vi "program seq..vi"(6 "IOList":T3, 7 "Cluster data":T5, 11 "Filepath":path=path "E:/My Project/2018-2019/Under development/Minda Ind. Switch -ID 144-145/Project/data/trail pro -12.txt") -> (0 "Error Out":errorcluster)   [LabVIEW 2015]
uses:
  Control PB/Active.ctl
  Control PB/deactive.ctl
  Control PB/output control.ctl
  Control PB/input control.ctl
  Control PB/timer.ctl
  Control PB/Remove list.ctl
  Control Button/Exit.ctl
  Control PB/Add_s.ctl
  Control PB/Delete_.ctl
  Control Button/Save.ctl
  Control PB/motor.ctl
  Control PB/Camera.ctl
  Control PB/Barcode.ctl
  Galobal variable_TI.vi
panel:
  out "Step List 4":string[](array[string])
  out "Step List 3":string[](array[string])
  in  "Barcode":T1
  in  "Camera":T2
  out "x <= y?":bool
  out "Cancel":bool
  out "Step List 2":string[](array[string])
  out "Pokayoka Result":cluster{"Sensor Name":string, "Boolean":bool}[](array[cluster])
  in  "Feed Back Channel":i32[](listbox)=[0]
  out "Input":bool[](array[boolean])
  out "Feature List (Out) 2":T4(array[cluster])
  out "error out 2":errorcluster
  in  "Control":bool
  out "Station No":string
  out "Model Name":string
  out "Machine Name":string
  in  "Motor":T6
  in  "Feature List":i32(listbox) caption="Steps List"
  in  "Deletefeature list":T7
  in  "Add feature list":T8
  in  "Deactive":T9
  in  "Active":T10
  in  "Program step":i32(listbox)
  in  "Remove Step":T11
  in  "Wait Time":u32=100 caption="Timer(ms)" max=600000 step=1
  in  "Timer":T12
  in  "Save":T13
  in  "stop":T14
  in  "op Add":T15
  in  "Input Add":T16
  out "Step List":string[](array[string])
  out "output cluster":T17
  in  "Analog":bool
  in  "Analog Input":i32[](listbox)=[0]
  in  "Control Channel":i32[](listbox)=[7]
  in  "Steps":T18(array[cluster])
  in  "Program mode":string="Data"
  out "error out":errorcluster
  out "Feature List (Out)":T19(array[cluster])
  # "Program Sequence Window"
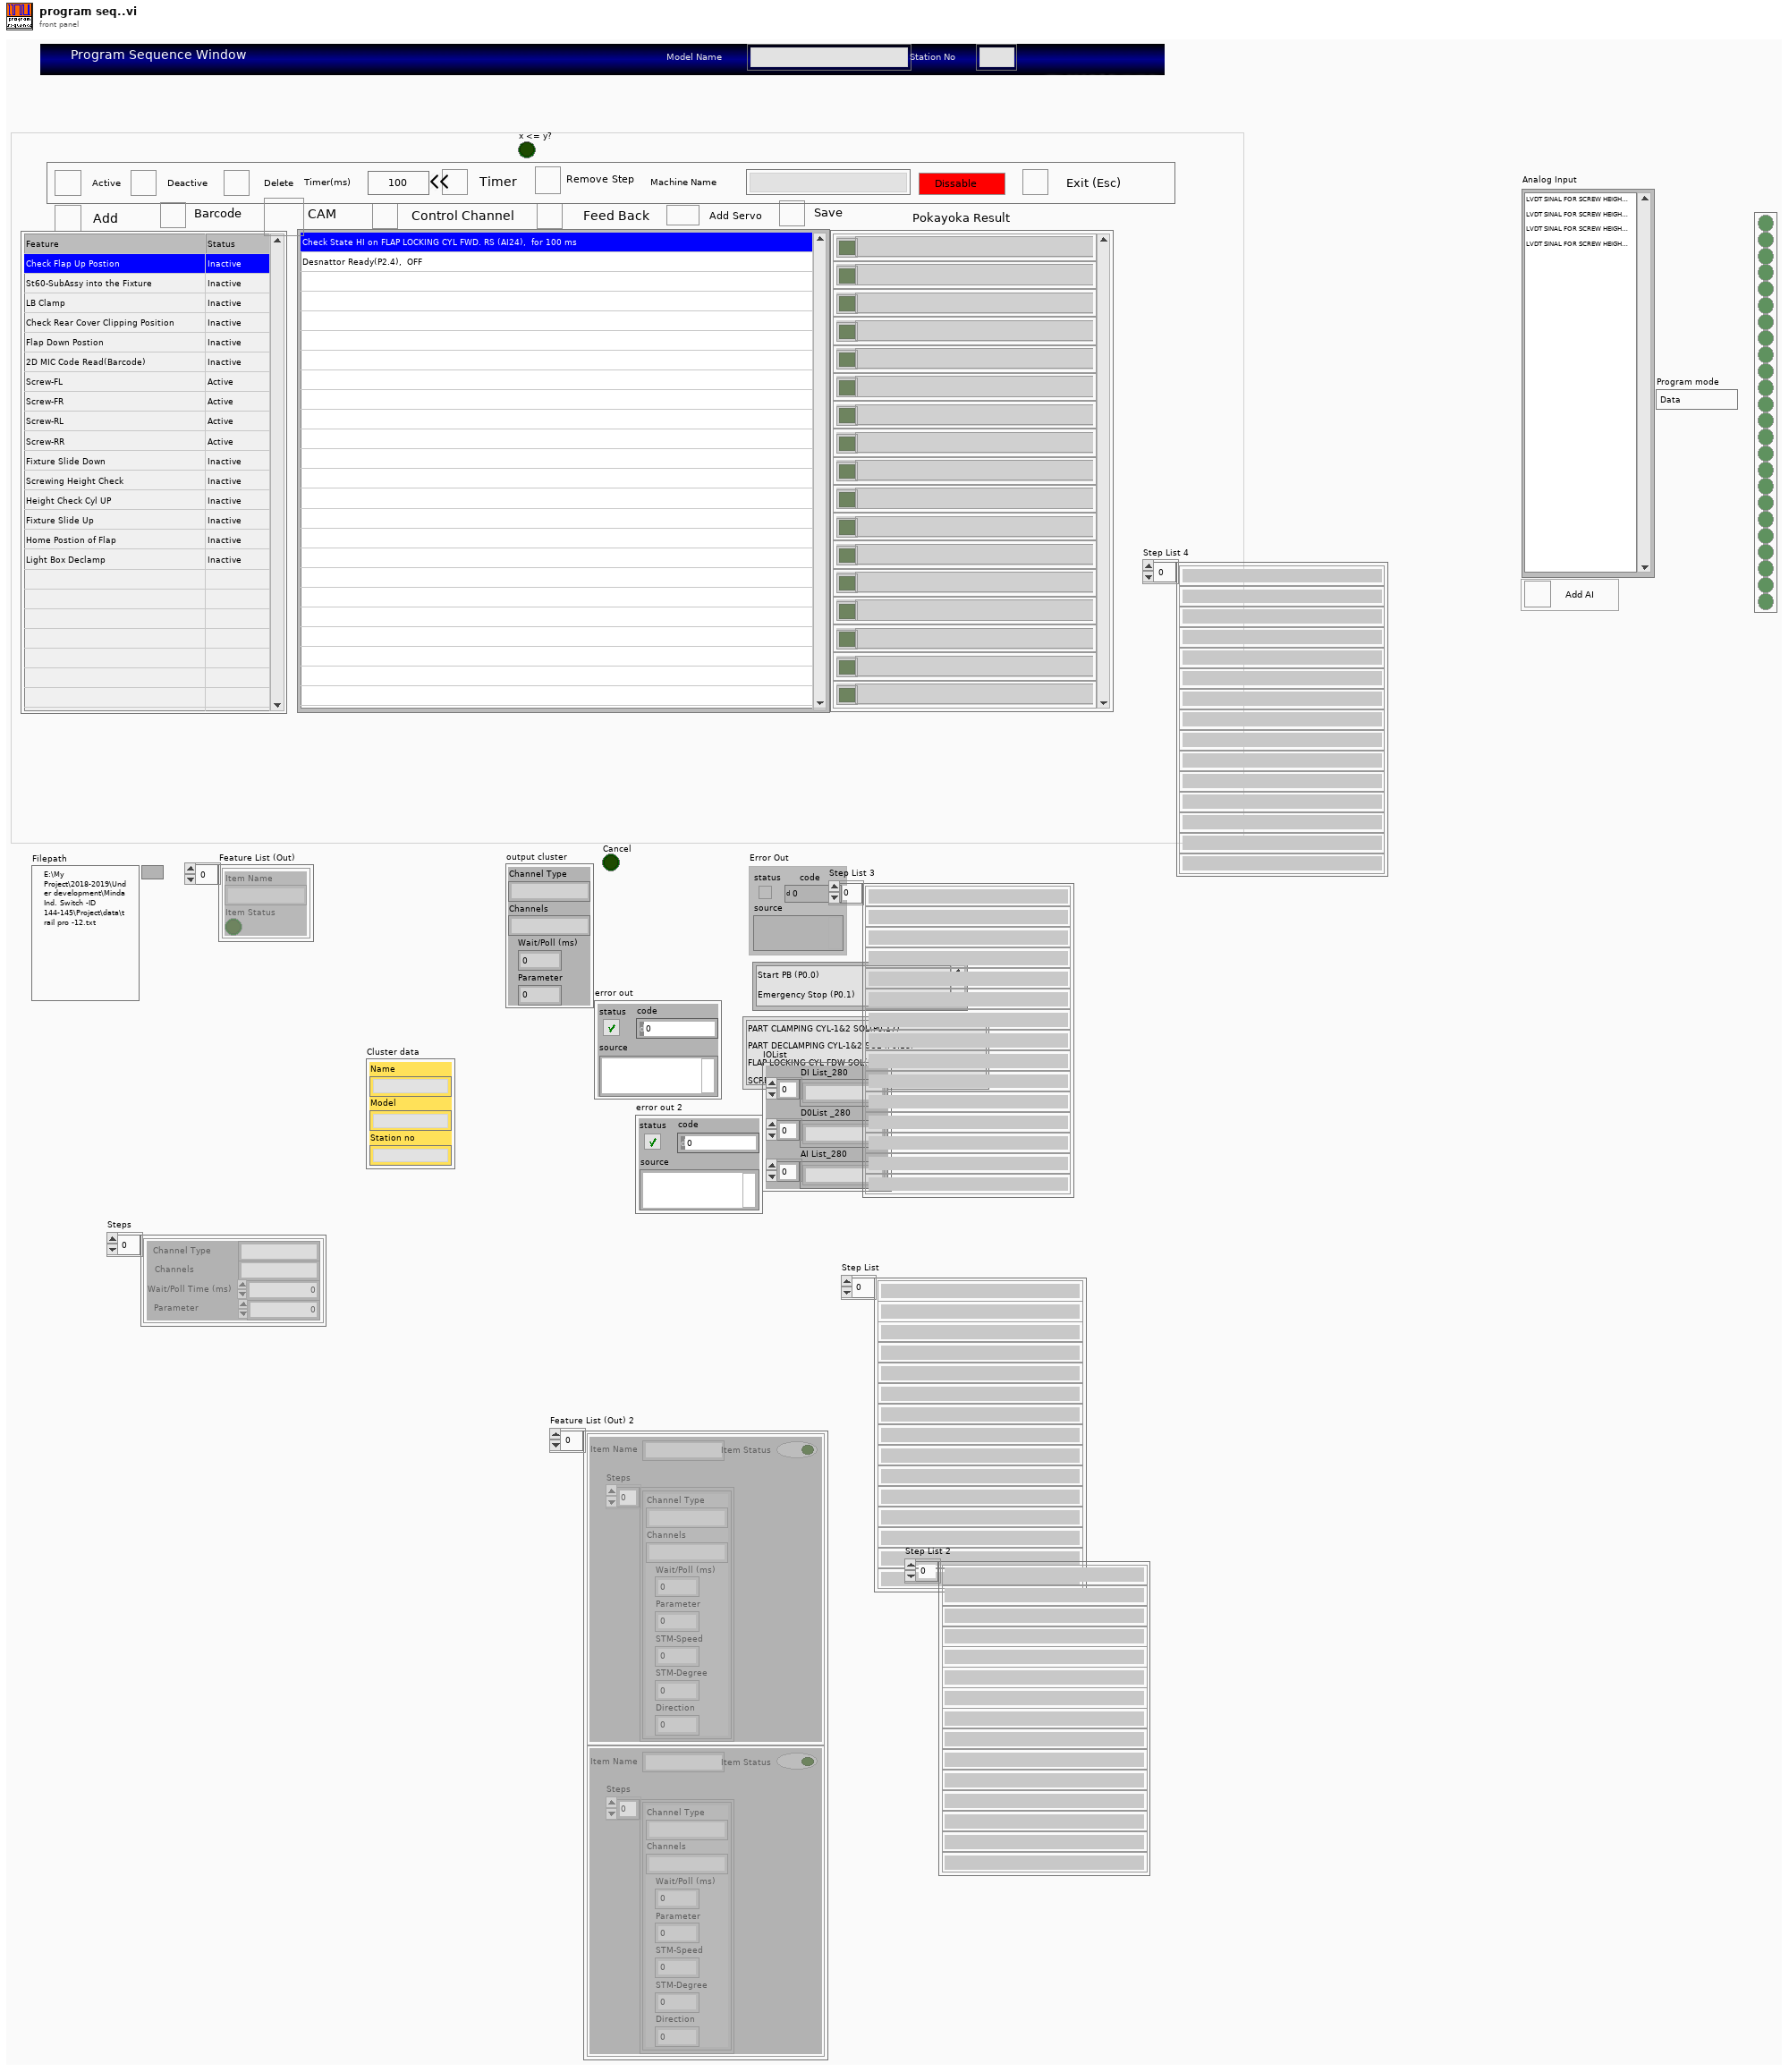
[diagram p1: front panel]
types:
  T1 = typedef "Barcode.ctl" = bool
  T2 = typedef "Camera.ctl" = bool
  T3 = cluster{"DI List_280":string[], "D0List _280":string[], "AI List_280":string[]}
  T4 = cluster{"Item Name":string, "Item Status":bool, "Steps":cluster{"Channel Type":string, "Channels":string, "Wait/Poll (ms)":u32, "Parameter":u8, "STM-Speed":i32, "STM-Degree":u32, "Direction":u8}[]}[]
  T5 = cluster{"Name":string, "Model":string, "Station no":string}
  T6 = typedef "motor.ctl" = bool
  T7 = typedef "Delete_.ctl" = bool
  T8 = typedef "Add_s.ctl" = bool
  T9 = typedef "deactive.ctl" = bool
  T10 = typedef "Active.ctl" = bool
  T11 = typedef "Remove list.ctl" = bool
  T12 = typedef "timer.ctl" = bool
  T13 = typedef "Save.ctl" = bool
  T14 = typedef "Exit.ctl" = bool
  T15 = typedef "output control.ctl" = bool
  T16 = typedef "input control.ctl" = bool
  T17 = cluster{"Channel Type":string, "Channels":string, "Wait/Poll (ms)":u32, "Parameter":u8}
  T18 = cluster{"Channel Type":string, "Channels":string, "Wait/Poll Time (ms)":u32, "Parameter":u8}[]
  T19 = cluster{"Item Name":string, "Item Status":bool}[]
  T20 = cluster{"Channel Type":string, "Channels":string, "Wait/Poll (ms)":u32, "Parameter":u8, "STM-Speed":i32, "STM-Degree":i32, "Direction":u8}
  T21 = cluster{"Item Name":string, "Item Status":bool, "Steps":cluster{"Channel Type":string, "Channels":string, "Wait/Poll (ms)":u32, "Parameter":u8, "STM-Speed":i32, "STM-Degree":u32, "Direction":u8}[]}
  T22 = cluster{"Channel Type":string, "Channels":string, "Wait/Poll (ms)":u32, "Parameter":u8, "STM-Speed":i32, "STM-Degree":u32, "Direction":u8}[]
  T23 = cluster{"Item Name":string, "Active":T10, "Steps":cluster{"Channel Type":string, "Channels":string, "Wait/Poll (ms)":u32, "Parameter":u8, "STM-Speed":i32, "STM-Degree":u32, "Direction":u8}[]}
  T24 = cluster{"Channel Type":string, "Channels":string, "Wait/Poll (ms)":u32, "Parameter":u8, "STM-Speed":i32, "STM-Degree":i32, "Direction":u8}[]
  T25 = cluster{"Feature name ":string, bool, cluster{"Channel Type":string, "Channels":string, "Wait/Poll (ms)":u32, "Parameter":u8, "STM-Speed":i32, "STM-Degree":i32, "Direction":u8}[]}
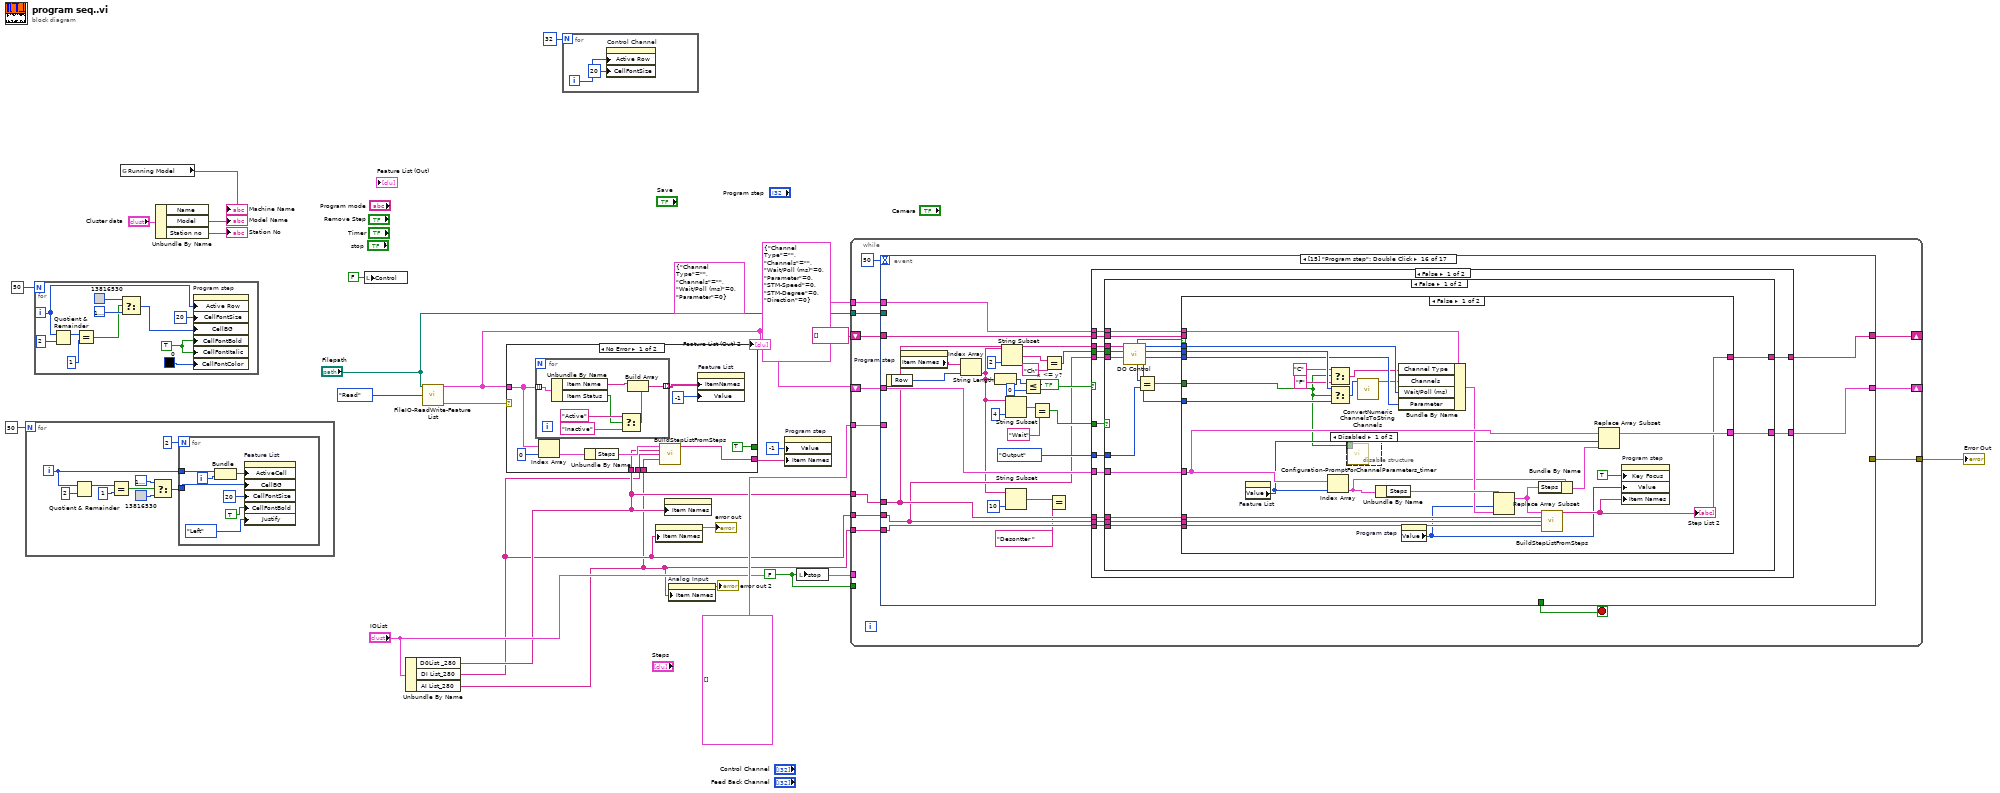
[diagram p0: block diagram]
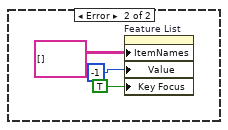
[diagram p2: hidden frame]
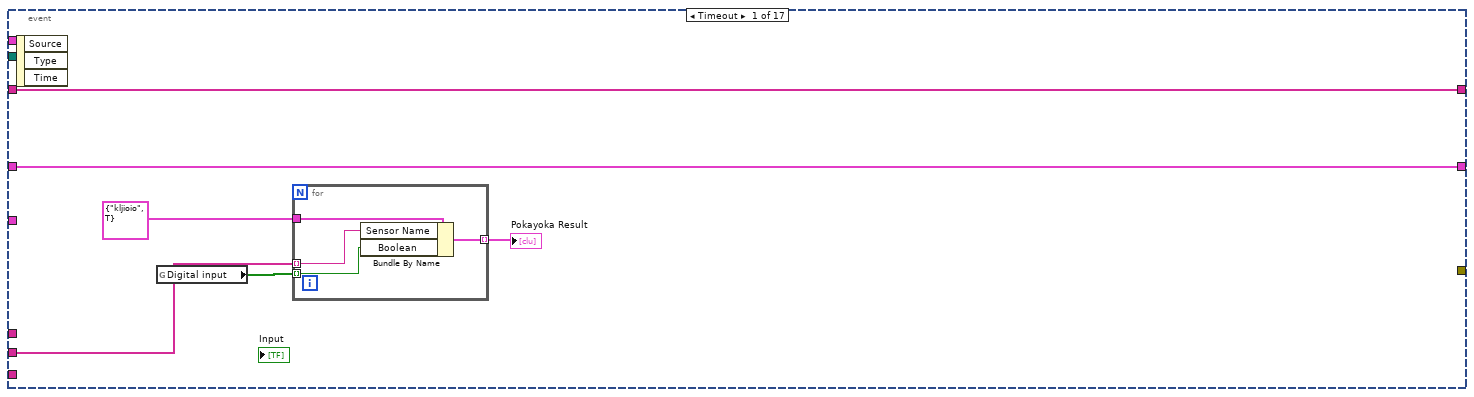
[diagram p3: hidden frame]
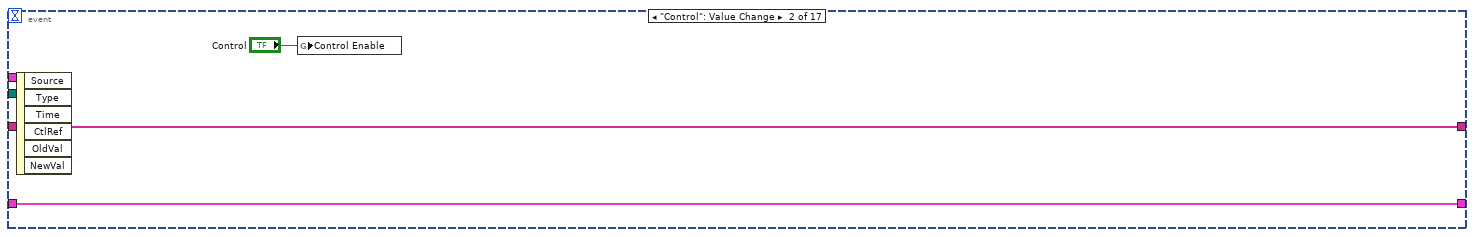
[diagram p4: hidden frame]
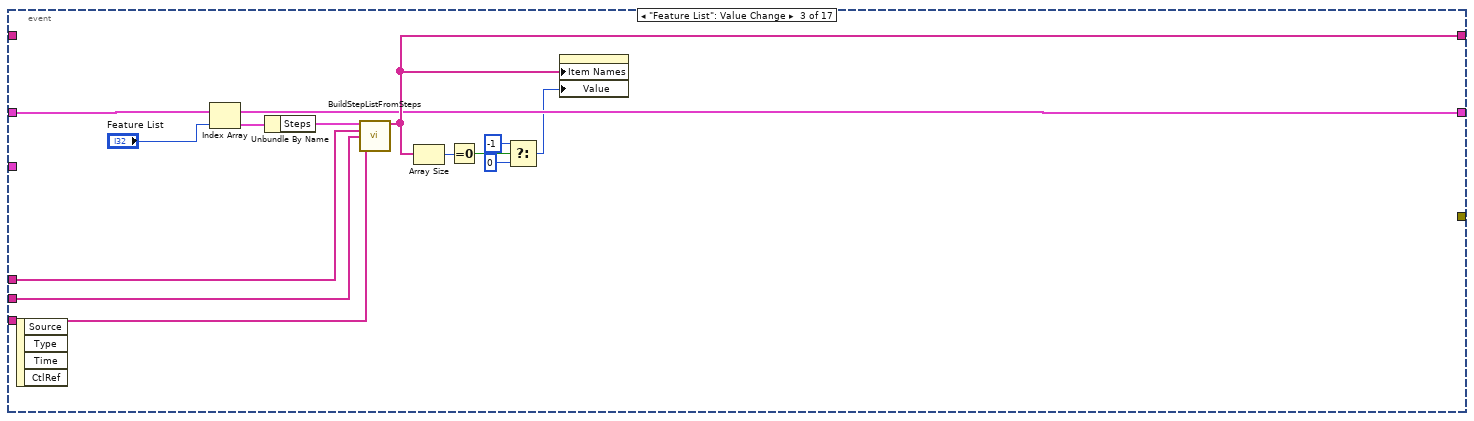
[diagram p5: hidden frame]
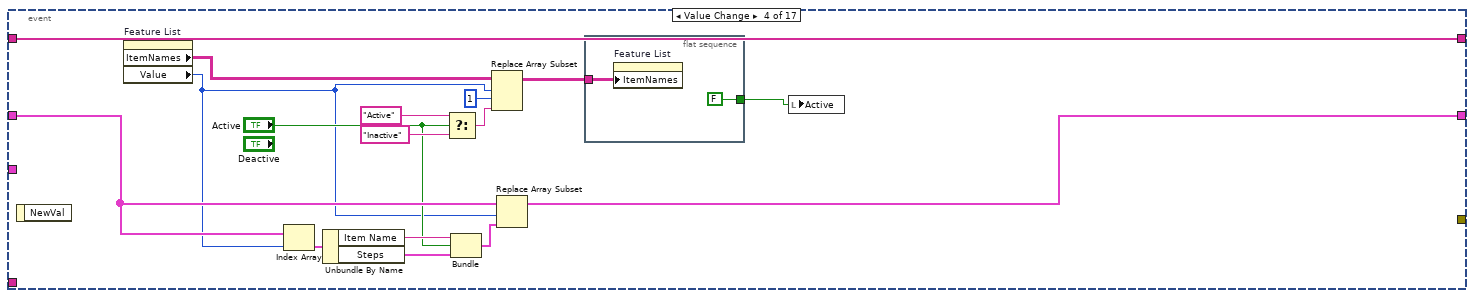
[diagram p6: hidden frame]
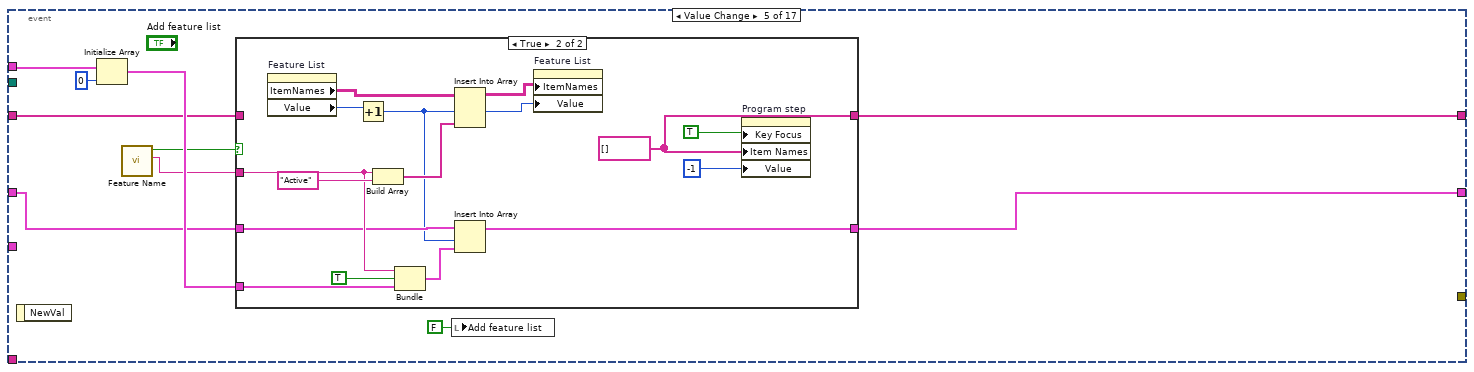
[diagram p7: hidden frame]
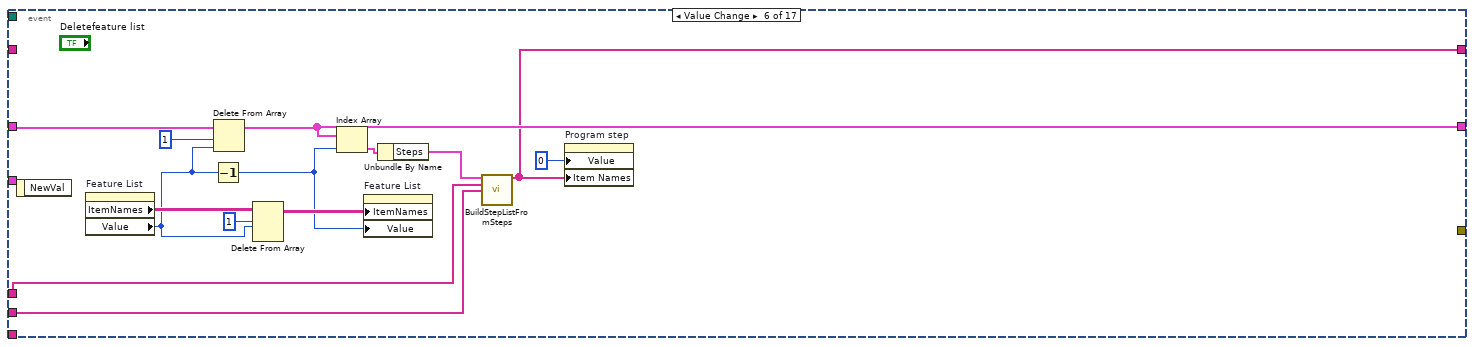
[diagram p9: hidden frame]
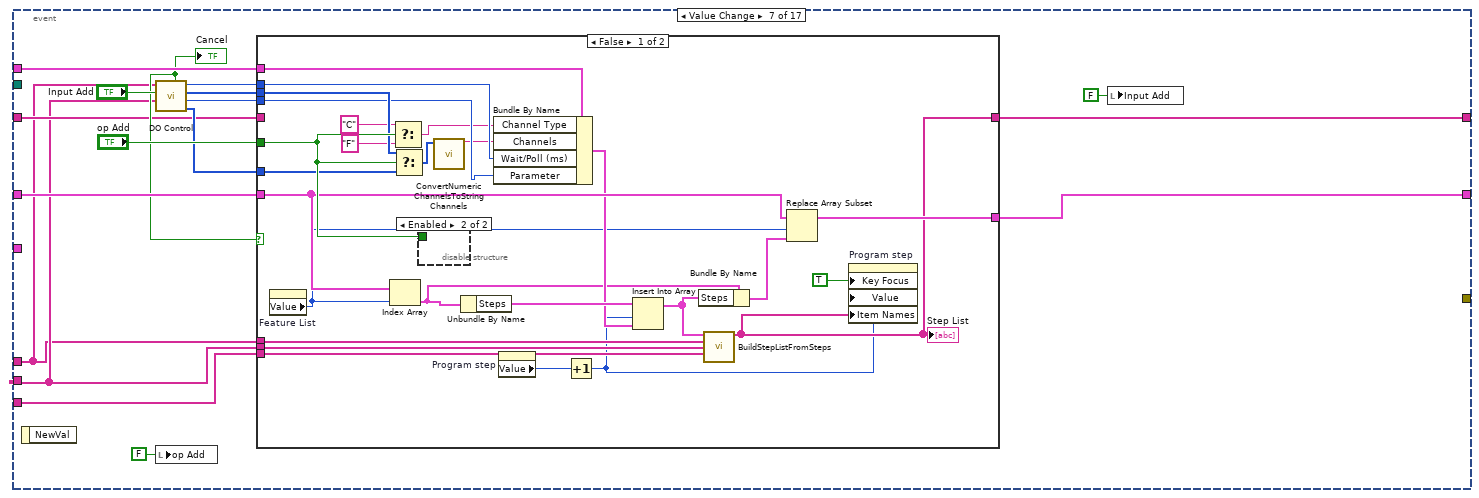
[diagram p10: hidden frame]
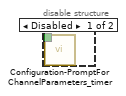
[diagram p11: hidden frame]
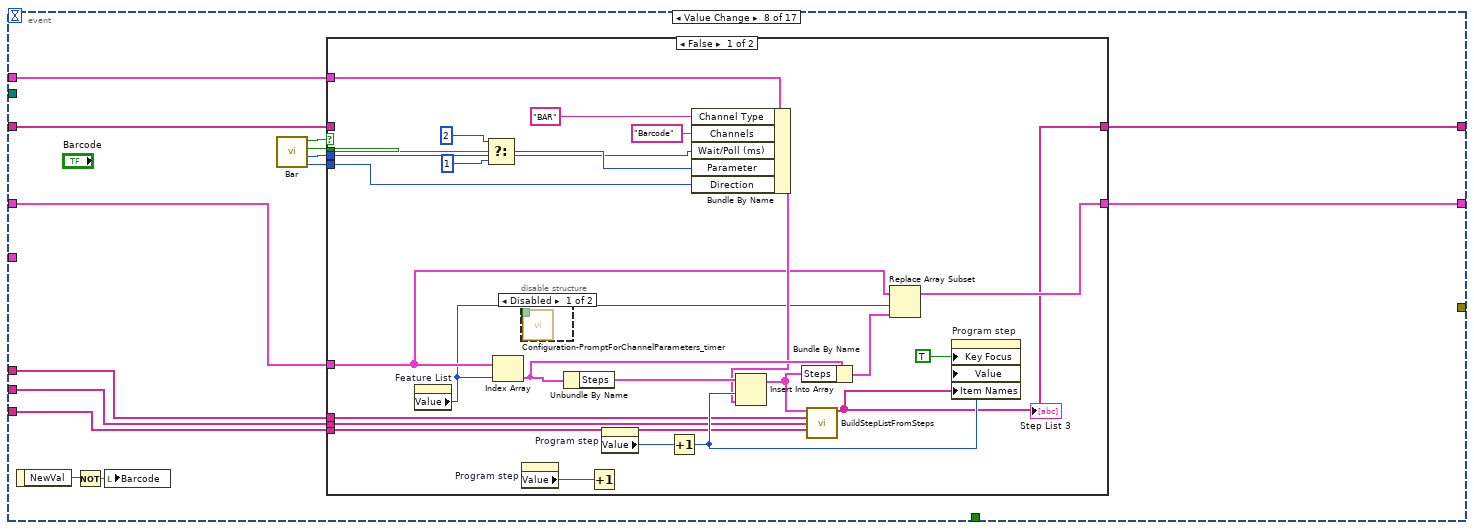
[diagram p13: hidden frame]
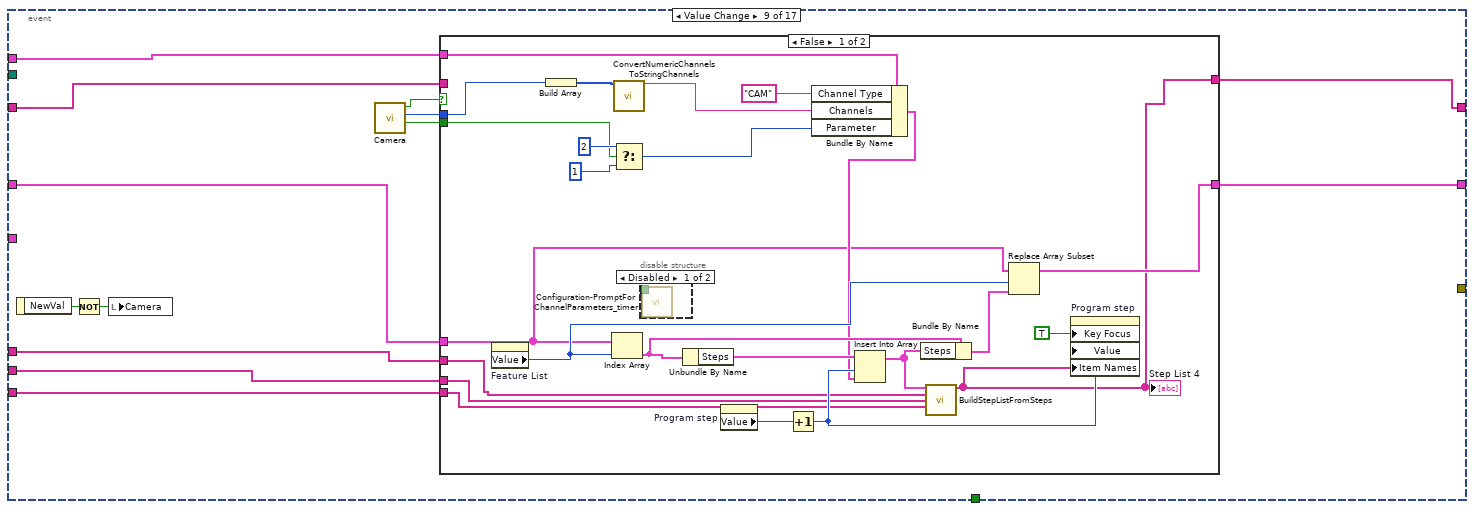
[diagram p16: hidden frame]
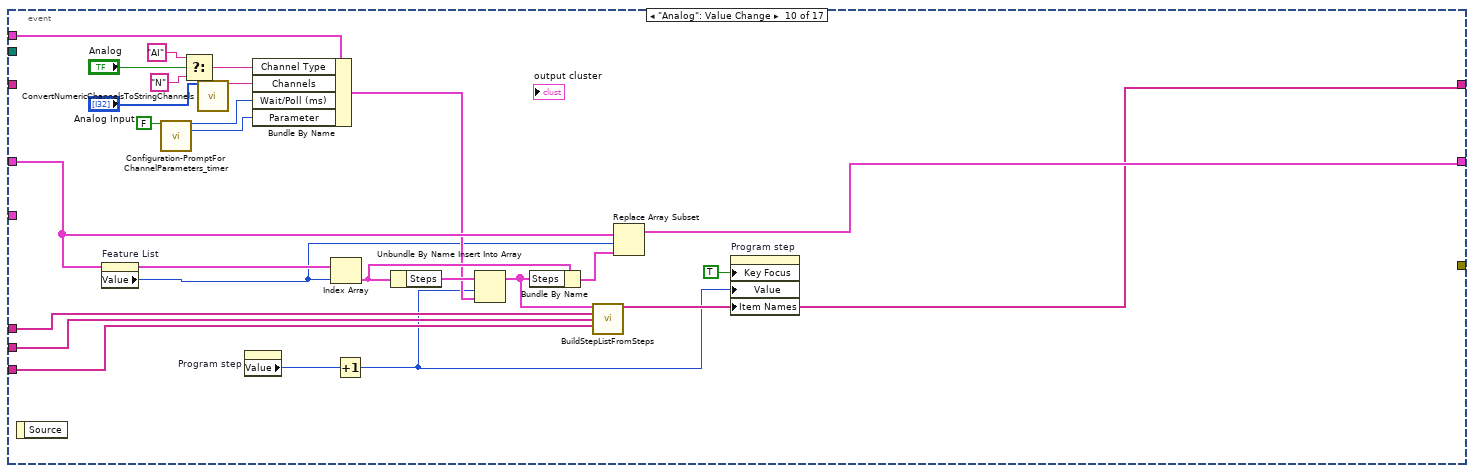
[diagram p19: hidden frame]
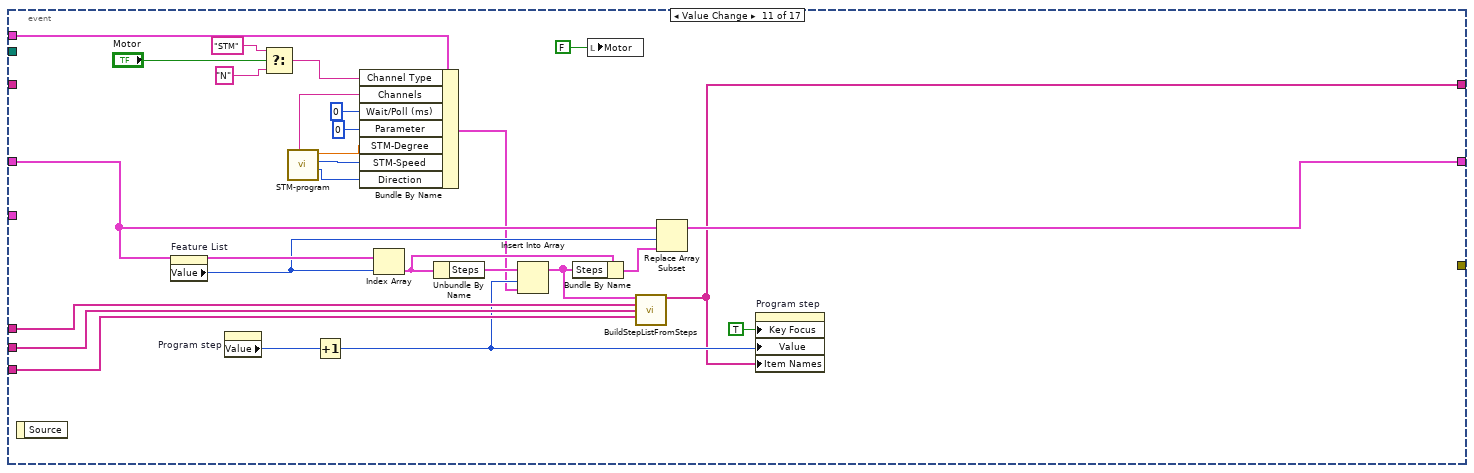
[diagram p20: hidden frame]
diagram:
  w9 = FALSE ("stop")
  (unwired) T17 {"Channel Type"="", "Channels"="", "Wait/Poll (ms)"=0, "Parameter"=0} ("Step")
  n1 = for {
    N: 50 -> [_]
    i -> [w33]
    n2 = Quotient & Remainder(x=w33, y=2) -> (x-y*floor(x/y)=w31:i32)  [unwired: 1 out]
    n3 = Equal?(x=w31, y=1) -> (x = y?=w29:bool)
    n4 = Select(t=u32 16777225 ("Color Box"), s=w29, f=u32 13816530 ("Color Box")) -> (s? t:f=w26:u32)
    n5 = for {
      N: 2 -> [_]
      tunnel: w33 -> [w41]
      tunnel: w26 -> [w38]
      i -> [w40]
      n6 = Bundle(w41, w40) -> (w39:cluster{i32, i32})  [unwired: 1 in]
      n7 = property on="Feature List" class="MCListbox (strict)"("ActiveCell"=w39, "CellBG"=w38, "CellFontSize"=u32 20 ("Active Cell:Cell Font:Size"), "CellFontBold"=TRUE ("Active Cell:Cell Font:Bold"), "Justify"=enum16{"Left", "Center", "Right"}."Left" ("Active Cell:Cell Justification")) -> ()  [unwired: 2 in, 2 out]
    }
  }
  n8 = for {
    N: 50 -> [_]
    i -> [w46]
    w43 = TRUE
    n9 = Quotient & Remainder(x=w46, y=2) -> (x-y*floor(x/y)=w49:i32)  [unwired: 1 out]
    n10 = Equal?(x=w49, y=1) -> (x = y?=w47:bool)
    n11 = Select(t=u32 13816530 ("Color Box"), s=w47, f=u32 16777226 ("Color Box")) -> (s? t:f=w44:u32)
    n12 = property on="Program step" class="LstBox (strict)"("Active Row"=w46, "CellFontSize"=u32 20 ("Active Row:Cell Font:Size"), "CellBG"=w44, "CellFontBold"=w43, "CellFontItalic"=w43, "CellFontColor"=u32 0 ("Color Box")) -> ()  [unwired: 2 in, 2 out]
  }
  n13 = global read "Galobal variable_TI.vi" "Running Model"() -> (→"Machine Name":string)
  n14 = Unbundle By Name("Cluster data") -> ("Model"=→"Model Name":string, "Station no"=→"Station No":string)  [unwired: 1 out]
  n15 = local write "Control"(FALSE ("Control")) -> ()
  n16 = Unbundle By Name("IOList") -> ("D0List _280"=w5:string[], "DI List_280"=w4:string[], "AI List_280"=w3:string[])
  n17 = call "FileIO-ReadWrite-FeatureList.vi"("Filepath"="Filepath", "Read/Write"=enum16{"Read", "Write"}."Read") -> ("Feature List (Out)"=w16:T4, "Error Out"=w20:errorcluster)  [unwired: 12 in]
  "Feature List (Out) 2" <- w16
  n18 = case shown="No Error" w20 {
    tunnel: w16 -> [w63 _]
    tunnel: w5 -> [w59 _]
    tunnel: w4 -> [w58 _]
    tunnel: w3 -> [w57 _]
    tunnel: [w56 _] -> w19
    tunnel: [TRUE ("Key Focus") _] -> _
    frame No Error {
      n19 = for {
        tunnel: w63 -> [w70] mode=indexing
        tunnel: [w64] -> w54 mode=indexing
        n20 = Unbundle By Name(w70) -> ("Item Name"=w66:string, "Item Status"=w67:bool)
        n21 = Select(t="Active", s=w67, f="Inactive") -> (s? t:f=w65:string)
        n22 = Build Array(w66, w65) -> (w64:string[])
      }
      n23 = Index Array(array=w63, index=0) -> (element=w61:T21)
      n24 = Unbundle By Name(w61) -> ("Steps"=w60:T22)
      n25 = call "BuildStepListFromSteps.vi"("Steps"=w60, "Control Channels"=w59, "Feedback Channels"=w58, "AI"=w57) -> ("Step List"=w56:string[])  [unwired: 11 in]
      n26 = property on="Feature List" class="MCListbox (strict)"("ItemNames"=w54, "Value"=-1 ("Feautre list")) -> ()  [unwired: 2 in, 2 out]
    }
    frame Error {
      n27 = property on="Feature List" class="MCListbox (strict)"("ItemNames"=string[][] [] ("Item Names"), "Value"=-1 ("Feautre list"), "Key Focus"=TRUE) -> ()  [unwired: 2 in, 2 out]
    }
  }
  n28 = for {
    N: 32 -> [_]
    i -> [w75]
    n29 = property on="Control Channel" class="LstBox (strict)"("Active Row"=w75, "CellFontSize"=u32 20 ("Active Row:Cell Font:Size")) -> ()  [unwired: 2 in, 2 out]
  }
  n30 = property on="Feed Back Channel" class="LstBox (strict)"("Item Names"=w4) -> (error out=→"error out":errorcluster)  [unwired: 2 in, 1 out]
  n31 = property on="Control Channel" class="LstBox (strict)"("Item Names"=w5) -> ()  [unwired: 2 in, 2 out]
  n32 = property on="Analog Input" class="LstBox (strict)"("Item Names"=w3) -> (error out=→"error out 2":errorcluster)  [unwired: 2 in, 1 out]
  n33 = property on="Program step" class="LstBox (strict)"("Value"=-1 ("Step feautre list"), "Item Names"=w19) -> ()  [unwired: 2 in, 2 out]
  n34 = local write "stop"(w9) -> ()
  n35 = while {
    shift-right: [w86] -> _
    shift-left: w16 -> [w77]
    tunnel: T20 {"Channel Type"="", "Channels"="", "Wait/Poll (ms)"=0, "Parameter"=0, "STM-Speed"=0, "STM-Degree"=0, "Direction"=0} ("Step") -> [w87]
    shift-right: [w85] -> _
    shift-left: string[] [] ("Step List") -> [w84]
    tunnel: w5 -> [w83]
    tunnel: w4 -> [w82]
    tunnel: [w81] -> w23
    tunnel: w3 -> [w80]
    tunnel: T4 [] ("Feature List (Out) 2") -> [w79]
    tunnel: "Filepath" -> [w78]
    tunnel: w9 -> [_]
    tunnel: "IOList" -> [_]
    stop <- w88 stop-if-true
    n36 = event shown="[15] \"Program step\": Double Click" {
      selector: _ -> [_ _ _ _ _ _ _ _ _ _ _ _ _ _ _ _ _]
      dyn-events: _ -> [_ _ _ _ _ _ _ _ _ _ _ _ _ _ _ _ _]
      timeout: 50 -> [_ _ _ _ _ _ _ _ _ _ _ _ _ _ _ _ _]
      tunnel: [_ _ _ _ _ _ _ _ _ _ _ _ _ _ TRUE ("stop") _ TRUE ("Discard?")] -> w88
      tunnel: w77 -> [w94 w100 w105 w122 w139 w171 w187 w228 w270 w311 w341 w362 w384 w393 w453 w478 w559]
      tunnel: w87 -> [_ _ _ _ w142 _ w190 w233 w274 w318 w346 w371 _ _ _ w479 _]
      tunnel: [w94 w100 w105 w120 w138 w170 w188 w227 w269 w306 w333 w361 w383 w395 w453 w476 w559] -> w86
      tunnel: [w93 w101 w108 w119 w135 w165 w186 w226 w268 w305 w332 w358 w378 w410 w452 w475 w560] -> w85
      tunnel: w84 -> [w93 w101 _ w119 w134 _ w177 w221 w265 _ _ _ _ _ w452 w474 w560]
      tunnel: w83 -> [_ _ w107 _ _ w167 w175 w229 w271 w308 w338 w360 w380 w412 _ w459 _]
      tunnel: w82 -> [w92 _ w106 _ _ w166 w176 w230 w272 w309 w337 w359 w379 w411 _ w458 _]
      tunnel: [_ _ _ _ _ _ _ _ _ _ _ _ _ w403 _ _ _] -> w81
      tunnel: w80 -> [_ _ w104 _ _ _ w185 w231 w273 w310 w336 w357 _ w404 _ w477 _]
      tunnel: w79 -> [_ _ _ _ _ _ _ _ _ _ _ _ _ w409 _ _ _]
      tunnel: w78 -> [_ _ _ _ _ _ _ _ _ _ _ _ _ w394 _ _ _]
      event Timeout {
        n37 = event-data() -> ()  [unwired: 1 in, 3 out]
        n38 = global read "Galobal variable_TI.vi" "Digital input"() -> (w89:bool[])
        n39 = for {
          tunnel: w92 -> [w97] mode=indexing
          tunnel: cluster{"Sensor Name":string, "Boolean":bool} {"Sensor Name"="kljioio", "Boolean"=TRUE} ("Cluster") -> [w98]
          tunnel: [w96] -> w90 mode=indexing
          tunnel: w89 -> [w95] mode=indexing
          n40 = Bundle By Name(cluster=w98, "Sensor Name"=w97, "Boolean"=w95) -> (w96:cluster{"Sensor Name":string, "Boolean":bool})
        }
        "Pokayoka Result" <- w90
      }
      event "Control": Value Change {
        n41 = event-data() -> ()  [unwired: 1 in, 6 out]
        n42 = global write "Galobal variable_TI.vi" "Control Enable"("Control") -> ()
      }
      event "Feature List": Value Change {
        n43 = event-data() -> ()  [unwired: 1 in, 4 out]
        n44 = Index Array(array=w105, index="Feature List") -> (element=w114:T21)
        n45 = Unbundle By Name(w114) -> ("Steps"=w113:T22)
        n46 = call "BuildStepListFromSteps.vi"("Steps"=w113, "Control Channels"=w107, "Feedback Channels"=w106, "AI"=w104) -> ("Step List"=w108:string[])  [unwired: 11 in]
        n47 = Array Size(array=w108) -> (size(s)=w110:i32)
        n48 = Equal To 0?(x=w110) -> (x = 0?=w112:bool)
        n49 = Select(t=-1 ("Step List"), s=w112, f=0 ("Step List")) -> (s? t:f=w103:i32)
        n50 = property on="Program step" class="LstBox (strict)"("Item Names"=w108, "Value"=w103) -> ()  [unwired: 2 in, 2 out]
      }
      event Value Change {
        n51 = event-data() -> ()  [unwired: 1 in, 1 out]
        n52 = property on="Feature List" class="MCListbox (strict)"() -> ("ItemNames"=w118:string[][], "Value"=w116:i32)  [unwired: 2 in, 2 out]
        n53 = Index Array(array=w122, index=w116) -> (element=w128:T21)
        n54 = Unbundle By Name(w128) -> ("Item Name"=w129:string, "Steps"=w130:T22)
        n55 = Select(t="Active", s="Active", f="Inactive" ("element")) -> (s? t:f=w125:string)
        n56 = Bundle("Item Name"=w129, "Active"="Active", "Steps"=w130) -> (w127:T23)  [unwired: 1 in]
        n57 = Replace Array Subset(array=w118, new element=w125, index (row)=w116, index (col)=1 ("disabled index (col)")) -> (w117:string[][])
        n58 = Replace Array Subset(array=w122, new element=w127, index=w116) -> (w120:T4)
        n59 = flat-sequence {
          tunnel: w117 -> [w132]
          tunnel: [T10 FALSE ("Active")] -> w115
          frame #0 {
            n60 = property on="Feature List" class="MCListbox (strict)"("ItemNames"=w132) -> ()  [unwired: 2 in, 2 out]
          }
        }
        n61 = local write "Active"(w115) -> ()
      }
      event Value Change {
        n62 = event-data() -> ()  [unwired: 1 in, 1 out]
        n63 = Initialize Array(w142, 0 ("dimension size")) -> (w140:T24)
        n64 = call "Feature Name.vi"() -> ("Feature name"=w136:string, "Out"=w137:bool)  [unwired: 10 in]
        n65 = case shown="True" w137 {
          tunnel: w140 -> [_ w158]
          tunnel: w139 -> [w144 w153]
          tunnel: [w144 w155] -> w138
          tunnel: w136 -> [_ w154]
          tunnel: [w143 w151] -> w135
          tunnel: w134 -> [w143 _]
          frame False {
          }
          frame True {
            w151 = string[] [] ("Item Names")
            n66 = property on="Feature List" class="MCListbox (strict)"() -> ("ItemNames"=w148:string[][], "Value"=w145:i32)  [unwired: 2 in, 2 out]
            n67 = Increment(x=w145) -> (x+1=w146:i32)
            n68 = Build Array(w154, "Active") -> (w149:string[])
            n69 = Bundle("Feature name"=w154, TRUE, w158) -> (w156:T25)  [unwired: 1 in]
            n70 = Insert Into Array(array=w148, index (row)=w146, new element=w149) -> (w147:string[][])  [unwired: 1 in]
            n71 = Insert Into Array(array=w153, index=w146, new element=w156) -> (w155:T4)
            n72 = property on="Feature List" class="MCListbox (strict)"("ItemNames"=w147, "Value"=w146) -> ()  [unwired: 2 in, 2 out]
            n73 = property on="Program step" class="LstBox (strict)"("Key Focus"=TRUE, "Item Names"=w151, "Value"=-1 ("Step feautre list")) -> ()  [unwired: 2 in, 2 out]
          }
        }
        n74 = local write "Add feature list"(FALSE ("Add feature list")) -> ()
      }
      event Value Change {
        n75 = event-data() -> ()  [unwired: 1 in, 1 out]
        n76 = property on="Feature List" class="MCListbox (strict)"() -> ("ItemNames"=w163:string[][], "Value"=w162:i32)  [unwired: 2 in, 2 out]
        n77 = Decrement(x=w162) -> (x-1=w160:i32)
        n78 = Delete From Array(array=w171, length=1, index=w162) -> (array with subset deleted=w170:T4)  [unwired: 1 out]
        n79 = Delete From Array(array=w163, length=1, index (row)=w162) -> (array with subset deleted=w161:string[][])  [unwired: 1 in, 1 out]
        n80 = Index Array(array=w170, index=w160) -> (element=w169:T21)
        n81 = property on="Feature List" class="MCListbox (strict)"("ItemNames"=w161, "Value"=w160) -> ()  [unwired: 2 in, 2 out]
        n82 = Unbundle By Name(w169) -> ("Steps"=w168:T22)
        n83 = call "BuildStepListFromSteps.vi"("Steps"=w168, "Control Channels"=w167, "Feedback Channels"=w166) -> ("Step List"=w165:string[])  [unwired: 12 in]
        n84 = property on="Program step" class="LstBox (strict)"("Value"=0 ("Step feautre list"), "Item Names"=w165) -> ()  [unwired: 2 in, 2 out]
      }
      event Value Change {
        n85 = event-data() -> ()  [unwired: 1 in, 1 out]
        n86 = call "DO Control.vi"("DI List_280"=w176, "s"="Input Add", "Control"=w175) -> ("Feedback"=w180:i32[], "Parameter (Out)"=w182:u8, "Control Channel"=w184:i32[], "Poll Time (Out)"=w183:u32, "Cancel"=w178:bool)  [unwired: 3 in, 1 out]
        "Cancel" <- w178
        n87 = local write "op Add"(T15 FALSE ("op Add")) -> ()
        n88 = case shown="False" w178 {
          tunnel: w190 -> [w216 _]
          tunnel: "op Add" -> [w215 _]
          tunnel: [w214 w219] -> w188
          tunnel: w187 -> [w213 w219]
          tunnel: w175 -> [w212 _]
          tunnel: w176 -> [w211 _]
          tunnel: [w210 w218] -> w186
          tunnel: w185 -> [w209 _]
          tunnel: w184 -> [w208 _]
          tunnel: w183 -> [w207 _]
          tunnel: w182 -> [w206 _]
          tunnel: w180 -> [w205 _]
          tunnel: w177 -> [_ w218]
          frame False {
            n89 = property on="Feature List" class="MCListbox (strict)"() -> ("Value"=w192:i32)  [unwired: 2 in, 2 out]
            n90 = Index Array(array=w213, index=w192) -> (element=w198:T21)
            n91 = Select(t="C", s=w215, f="F") -> (s? t:f=w202:string)
            n92 = Select(t=w208, s=w215, f=w205) -> (s? t:f=w191:i32[])
            n93 = disable-structure shown="Enabled" {
              disable-tunnel: w215 -> [w217 _]
              frame Disabled {
                n94 = call "Configuration-PromptForChannelParameters_timer.vi"("Control/Feedback\n(Default: False = Feedback)"=w217) -> ()  [unwired: 13 in, 2 out]
              }
              frame Enabled {
              }
            }
            n95 = call "ConvertNumericChannelsToStringChannels.vi"("Channels (In)"=w191) -> ("Channels (A:B:C:D...) (Out)"=w201:string)  [unwired: 14 in]
            n96 = Unbundle By Name(w198) -> ("Steps"=w200:T22)
            n97 = Bundle By Name(cluster=w216, "Channel Type"=w202, "Channels"=w201, "Wait/Poll (ms)"=w207, "Parameter"=w206) -> (w199:T20)
            n98 = property on="Program step" class="LstBox (strict)"() -> ("Value"=w193:i32)  [unwired: 2 in, 2 out]
            n99 = Increment(x=w193) -> (x+1=w194:i32)
            n100 = Insert Into Array "Insert Into Array"(array=w200, index=w194, new element=w199) -> (w196:T22)
            n101 = Bundle By Name(cluster=w198, "Steps"=w196) -> (w197:T21)
            n102 = call "BuildStepListFromSteps.vi"("Steps"=w196, "Control Channels"=w212, "Feedback Channels"=w211, "AI"=w209) -> ("Step List"=w210:string[])  [unwired: 11 in]
            "Step List" <- w210
            n103 = Replace Array Subset(array=w213, new element=w197, index=w192) -> (w214:T4)
            n104 = property on="Program step" class="LstBox (strict)"("Key Focus"=TRUE, "Value"=w194, "Item Names"=w210) -> ()  [unwired: 2 in, 2 out]
          }
          frame True {
          }
        }
        n105 = local write "Input Add"(T16 FALSE ("Input Add")) -> ()
      }
      event Value Change {
        n106 = event-data() -> ("NewVal"=w224:T1)  [unwired: 1 in]
        n107 = Not(x=w224) -> (.not. x?=w223:T1)
        n108 = local write "Barcode"(w223) -> ()
        n109 = call "Bar.vi"() -> ("Numeric"=w220:i32, "Time Out Value"=w225:u8, "Barcode Scane"=w232:bool, "Out"=w222:bool)  [unwired: 8 in]
        n110 = case shown="False" w222 {
          tunnel: w233 -> [w258 _]
          tunnel: w232 -> [w255 _]
          tunnel: w231 -> [w242 _]
          tunnel: w230 -> [w241 _]
          tunnel: w229 -> [w240 _]
          tunnel: w228 -> [w239 w260]
          tunnel: [w238 w260] -> w227
          tunnel: [w237 w261] -> w226
          tunnel: w225 -> [w236 _]
          tunnel: w221 -> [_ w261]
          tunnel: w220 -> [w234 _]
          frame False {
            n111 = property on="Feature List" class="MCListbox (strict)"() -> ("Value"=w235:i32)  [unwired: 2 in, 2 out]
            n112 = Select(t=2, s=w255, f=1) -> (s? t:f=w252:i32)
            n113 = Index Array(array=w239, index=w235) -> (element=w250:T21)
            n114 = disable-structure shown="Disabled" {
              disable-tunnel: _ -> [w259 _]
              frame Disabled {
                n115 = call "Configuration-PromptForChannelParameters_timer.vi"("Control/Feedback\n(Default: False = Feedback)"=w259) -> ()  [unwired: 13 in, 2 out]
              }
              frame Enabled {
              }
            }
            n116 = property on="Program step" class="LstBox (strict)"() -> ("Value"=w244:i32)  [unwired: 2 in, 2 out]
            n117 = Unbundle By Name(w250) -> ("Steps"=w251:T22)
            n118 = Increment(x=w244) -> ()  [unwired: 1 out]
            n119 = property on="Program step" class="LstBox (strict)"() -> ("Value"=w245:i32)  [unwired: 2 in, 2 out]
            n120 = Increment(x=w245) -> (x+1=w246:i32)
            n121 = Bundle By Name(cluster=w258, "Channel Type"="BAR", "Channels"="Barcode", "Wait/Poll (ms)"=w236, "Parameter"=w252, "Direction"=w234) -> (w243:T20)
            n122 = Insert Into Array "Insert Into Array"(array=w251, index=w246, new element=w243) -> (w248:T22)
            n123 = Bundle By Name(cluster=w250, "Steps"=w248) -> (w249:T21)
            n124 = call "BuildStepListFromSteps.vi"("Steps"=w248, "Control Channels"=w240, "Feedback Channels"=w241, "AI"=w242) -> ("Step List"=w237:string[])  [unwired: 11 in]
            "Step List 3" <- w237
            n125 = Replace Array Subset(array=w239, new element=w249, index=w235) -> (w238:T4)
            n126 = property on="Program step" class="LstBox (strict)"("Key Focus"=TRUE, "Value"=w246, "Item Names"=w237) -> ()  [unwired: 2 in, 2 out]
          }
          frame True {
          }
        }
      }
      event Value Change {
        n127 = event-data() -> ("NewVal"=w262:T2)  [unwired: 1 in]
        n128 = Not(x=w262) -> (.not. x?=w263:T2)
        n129 = local write "Camera"(w263) -> ()
        n130 = call "Camera.vi"() -> ("Camera 2"=w266:bool, "Feature list  3"=w267:i32, "Out"=w264:bool)  [unwired: 9 in]
        n131 = case shown="False" w264 {
          tunnel: w274 -> [w286 _]
          tunnel: w273 -> [w285 _]
          tunnel: w272 -> [w284 _]
          tunnel: w271 -> [w283 _]
          tunnel: w270 -> [w282 w300]
          tunnel: [w281 w300] -> w269
          tunnel: [w280 w301] -> w268
          tunnel: w267 -> [w277 _]
          tunnel: w266 -> [w279 _]
          tunnel: w265 -> [_ w301]
          frame False {
            n132 = property on="Feature List" class="MCListbox (strict)"() -> ("Value"=w288:i32)  [unwired: 2 in, 2 out]
            n133 = Build Array(w277) -> (w276:i32[])
            n134 = Index Array(array=w282, index=w288) -> (element=w294:T21)
            n135 = call "ConvertNumericChannelsToStringChannels.vi"("Channels (In)"=w276) -> ("Channels (A:B:C:D...) (Out)"=w275:string)  [unwired: 14 in]
            n136 = Select(t=2, s=w279, f=1) -> (s? t:f=w278:i32)
            n137 = disable-structure shown="Disabled" {
              disable-tunnel: _ -> [w299 _]
              frame Disabled {
                n138 = call "Configuration-PromptForChannelParameters_timer.vi"("Control/Feedback\n(Default: False = Feedback)"=w299) -> ()  [unwired: 13 in, 2 out]
              }
              frame Enabled {
              }
            }
            n139 = Unbundle By Name(w294) -> ("Steps"=w295:T22)
            n140 = property on="Program step" class="LstBox (strict)"() -> ("Value"=w289:i32)  [unwired: 2 in, 2 out]
            n141 = Increment(x=w289) -> (x+1=w290:i32)
            n142 = Bundle By Name(cluster=w286, "Channel Type"="CAM", "Channels"=w275, "Parameter"=w278) -> (w287:T20)
            n143 = Insert Into Array "Insert Into Array"(array=w295, index=w290, new element=w287) -> (w292:T22)
            n144 = Bundle By Name(cluster=w294, "Steps"=w292) -> (w293:T21)
            n145 = call "BuildStepListFromSteps.vi"("Steps"=w292, "Control Channels"=w283, "Feedback Channels"=w284, "AI"=w285) -> ("Step List"=w280:string[])  [unwired: 11 in]
            "Step List 4" <- w280
            n146 = Replace Array Subset(array=w282, new element=w293, index=w288) -> (w281:T4)
            n147 = property on="Program step" class="LstBox (strict)"("Key Focus"=TRUE, "Value"=w290, "Item Names"=w280) -> ()  [unwired: 2 in, 2 out]
          }
          frame True {
          }
        }
      }
      event "Analog": Value Change {
        n148 = event-data() -> ()  [unwired: 1 in, 1 out]
        n149 = property on="Feature List" class="MCListbox (strict)"() -> ("Value"=w302:i32)  [unwired: 2 in, 2 out]
        n150 = call "Configuration-PromptForChannelParameters_timer.vi"("Control/Feedback\n(Default: False = Feedback)"=FALSE ("Control/Feedback\n(Default: False = Feedback)")) -> ("Poll Time (Out)"=w322:u32, "Parameter (Out)"=w321:u8)  [unwired: 13 in]
        n151 = Select(t="AI", s="Analog", f="N") -> (s? t:f=w324:string)
        n152 = call "ConvertNumericChannelsToStringChannels.vi"("Channels (In)"="Analog Input") -> ("Channels (A:B:C:D...) (Out)"=w323:string)  [unwired: 14 in]
        n153 = property on="Program step" class="LstBox (strict)"() -> ("Value"=w312:i32)  [unwired: 2 in, 2 out]
        n154 = Bundle By Name(cluster=w318, "Channel Type"=w324, "Channels"=w323, "Wait/Poll (ms)"=w322, "Parameter"=w321) -> (w307:T20)
        n155 = Index Array(array=w311, index=w302) -> (element=w316:T21)
        n156 = Increment(x=w312) -> (x+1=w303:i32)
        n157 = Unbundle By Name(w316) -> ("Steps"=w317:T22)
        n158 = Insert Into Array(array=w317, index=w303, new element=w307) -> (w314:T22)
        n159 = Bundle By Name(cluster=w316, "Steps"=w314) -> (w315:T21)
        n160 = call "BuildStepListFromSteps.vi"("Steps"=w314, "Control Channels"=w308, "Feedback Channels"=w309, "AI"=w310) -> ("Step List"=w305:string[])  [unwired: 11 in]
        n161 = Replace Array Subset(array=w311, new element=w315, index=w302) -> (w306:T4)
        n162 = property on="Program step" class="LstBox (strict)"("Key Focus"=TRUE, "Value"=w303, "Item Names"=w305) -> ()  [unwired: 2 in, 2 out]
      }
      event Value Change {
        n163 = event-data() -> ()  [unwired: 1 in, 1 out]
        n164 = property on="Feature List" class="MCListbox (strict)"() -> ("Value"=w340:i32)  [unwired: 2 in, 2 out]
        n165 = property on="Program step" class="LstBox (strict)"() -> ("Value"=w339:i32)  [unwired: 2 in, 2 out]
        n166 = Select(t="STM", s="Motor", f="N") -> (s? t:f=w351:string)
        n167 = call "STM-program.vi"() -> ("OutDir"=w350:i32, "Out Speed"=w348:i32, "Out Degree"=w349:dbl, "Channels (A:B:C:D...) (Out)"=w328:string)  [unwired: 7 in, 1 out]
        n168 = Increment(x=w339) -> (x+1=w334:i32)
        n169 = Bundle By Name(cluster=w346, "Channel Type"=w351, "Channels"=w328, "Wait/Poll (ms)"=u32 0, "Parameter"=u8 0, "STM-Degree"=w349, "STM-Speed"=w348, "Direction"=w350) -> (w331:T20)
        n170 = Index Array(array=w341, index=w340) -> (element=w344:T21)
        n171 = Unbundle By Name(w344) -> ("Steps"=w345:T22)
        n172 = Insert Into Array(array=w345, index=w334, new element=w331) -> (w342:T22)
        n173 = Bundle By Name(cluster=w344, "Steps"=w342) -> (w343:T21)
        n174 = local write "Motor"(FALSE ("Motor")) -> ()
        n175 = call "BuildStepListFromSteps.vi"("Steps"=w342, "Control Channels"=w338, "Feedback Channels"=w337, "AI"=w336) -> ("Step List"=w332:string[])  [unwired: 11 in]
        n176 = Replace Array Subset(array=w341, new element=w343, index=w340) -> (w333:T4)
        n177 = property on="Program step" class="LstBox (strict)"("Key Focus"=TRUE, "Value"=w334, "Item Names"=w332) -> ()  [unwired: 2 in, 2 out]
      }
      event Value Change {
        n178 = event-data() -> ()  [unwired: 1 in, 1 out]
        n179 = property on="Feature List" class="MCListbox (strict)"() -> ("Value"=w354:i32)  [unwired: 2 in, 2 out]
        n180 = Index Array(array=w362, index=w354) -> (element=w365:T21)
        n181 = Bundle By Name(cluster=w371, "Channel Type"="N", "Wait/Poll (ms)"="Wait Time") -> (w367:T20)
        n182 = Unbundle By Name(w365) -> ("Steps"=w366:T22)
        n183 = property on="Program step" class="LstBox (strict)"() -> ("Value"=w368:i32)  [unwired: 2 in, 2 out]
        n184 = Increment(x=w368) -> (x+1=w355:i32)
        n185 = Insert Into Array(array=w366, index=w355, new element=w367) -> (w363:T22)
        n186 = Bundle By Name(cluster=w365, "Steps"=w363) -> (w364:T21)
        n187 = call "BuildStepListFromSteps.vi"("Steps"=w363, "Control Channels"=w360, "Feedback Channels"=w359, "AI"=w357) -> ("Step List"=w358:string[])  [unwired: 11 in]
        n188 = property on="Program step" class="LstBox (strict)"("Item Names"=w358, "Value"=w355, "Key Focus"=TRUE) -> ()  [unwired: 2 in, 2 out]
        n189 = Replace Array Subset(array=w362, new element=w364, index=w354) -> (w361:T4)
      }
      event Value Change {
        n190 = event-data() -> ()  [unwired: 1 in, 2 out]
        n191 = property on="Feature List" class="MCListbox (strict)"() -> ("Value"=w373:i32)  [unwired: 2 in, 2 out]
        n192 = Index Array(array=w384, index=w373) -> (element=w390:T21)
        n193 = property on="Program step" class="LstBox (strict)"() -> ("Value"=w372:i32)  [unwired: 2 in, 2 out]
        n194 = Unbundle By Name(w390) -> ("Item Name"=w388:string, "Item Status"=w387:bool, "Steps"=w386:T22)
        n195 = Equal?(x=w372, y=-1) -> (x = y?=w376:bool)
        n196 = Select(t=0 ("y"), s=w376, f=w372) -> (s? t:f=w374:i32)
        n197 = Delete From Array(array=w386, length=1, index=w374) -> (array with subset deleted=w382:T22)  [unwired: 1 out]
        n198 = Bundle("Item Name"=w388, "Item Status"=w387, "Steps"=w382) -> (w385:T21)  [unwired: 1 in]
        n199 = call "BuildStepListFromSteps.vi"("Steps"=w382, "Control Channels"=w380, "Feedback Channels"=w379) -> ("Step List"=w378:string[])  [unwired: 12 in]
        n200 = Replace Array Subset(array=w384, new element=w385, index=w373) -> (w383:T4)
        n201 = property on="Program step" class="LstBox (strict)"("Item Names"=w378, "Value"=w374, "Key Focus"=TRUE) -> ()  [unwired: 2 in, 2 out]
      }
      event Value Change {
        n202 = event-data() -> ()  [unwired: 1 in, 1 out]
        n203 = for {
          tunnel: w393 -> [w440] mode=indexing
          tunnel: [w435] -> w401 mode=indexing
          shift-right: [w434] -> w402
          shift-left: w409 -> [w437]
          n204 = Unbundle By Name(w440) -> ("Steps"=w441:T22, "Item Name"=w439:string, "Item Status"=w438:bool)
          n205 = Array Size(array=w441) -> (size(s)=w436:i32)
          n206 = case shown="Default" w436 {
            tunnel: w441 -> [_ w448]
            tunnel: w439 -> [_ w450]
            tunnel: w438 -> [_ w449]
            tunnel: [w443 w446] -> w434
            tunnel: w437 -> [w443 w444]
            tunnel: [FALSE TRUE] -> w435
            frame 0 {
            }
            frame Default {
              n207 = Bundle("Item Name"=w450, "Item Status"=w449, "Steps"=w448) -> (w445:T21)  [unwired: 1 in]
              n208 = Build Array (concatenate)(w444, w445) -> (w446:T4)
            }
          }
        }
        n209 = And Array Elements(Boolean array=w401) -> (logical AND=w400:bool)
        n210 = case shown="True" w400 {
          tunnel: [w413 w415] -> w395
          tunnel: w394 -> [_ w423]
          tunnel: [_ w421] -> w403
          tunnel: w402 -> [_ w416]
          tunnel: enum16{"Read", "Write"}."Write" ("Read/Write") -> [_ w422]
          tunnel: "Feature List successfully saved." -> [_ w420]
          tunnel: "Error in saving Feature List." -> [_ w419]
          tunnel: "Can't save Feature List as at least one feature doesn't have steps.\nPlease check." ("message") -> [w414 w418]
          tunnel: w393 -> [w413 _]
          frame False {
            n211 = One Button Dialog(message=w414) -> ()  [unwired: 1 in, 1 out]
          }
          frame True {
            n212 = call "FileIO-ReadWrite-FeatureList.vi"("Filepath"=w423, "Feature List (In)"=w416, "Read/Write"=w422) -> ("Feature List (Out)"=w415:T4, "Error Out"=w421:errorcluster)  [unwired: 11 in]
            n213 = case shown="Error" w421 {
              tunnel: w420 -> [w424 _]
              tunnel: w419 -> [_ w425]
              tunnel: w418 -> [_ _]
              tunnel: [w424 w425] -> w417
              frame No Error {
              }
              frame Error {
              }
            }
            n214 = One Button Dialog(message=w417) -> ()  [unwired: 1 in, 1 out]
          }
        }
        n215 = disable-structure shown="Enabled" {
          frame Disabled {
            n216 = call "Program seq path.vi"() -> ()  [unwired: 11 in, 1 out]
          }
          frame Enabled {
          }
        }
        n217 = Index Array(array=w395, index=0) -> (element=w407:T21)
        n218 = Unbundle By Name(w407) -> ("Steps"=w406:T22)
        n219 = for {
          tunnel: [w432] -> w392 mode=indexing
          tunnel: w395 -> [w427] mode=indexing
          tunnel: [w426] -> _
          i -> [w426]
          n220 = Unbundle By Name(w427) -> ("Item Name"=w433:string, "Item Status"=w431:bool)
          n221 = Select(t="Active", s=w431, f="Inactive") -> (s? t:f=w428:string)
          n222 = Build Array(w433, w428) -> (w432:string[])
        }
        n223 = call "BuildStepListFromSteps.vi"("Steps"=w406, "Control Channels"=w412, "Feedback Channels"=w411, "AI"=w404) -> ("Step List"=w410:string[])  [unwired: 11 in]
        n224 = property on="Program step" class="LstBox (strict)"("Item Names"=w410, "Value"=0 ("Step feautre list")) -> ()  [unwired: 2 in, 2 out]
        n225 = property on="Feature List" class="MCListbox (strict)"("ItemNames"=w392, "Value"=0 ("Feautre list")) -> ()  [unwired: 2 in, 2 out]
      }
      event Value Change {
        n226 = event-data() -> ()  [unwired: 1 in, 1 out]
      }
      event "Program step": Double Click {
        n227 = event-data() -> ("Row"=w472:i32)  [unwired: 1 in]
        n228 = property on="Program step" class="LstBox (strict)"() -> ("Item Names"=w473:string[])  [unwired: 2 in, 2 out]
        n229 = Index Array(array=w473, index=w472) -> (element=w456:string)
        n230 = String Length(string=w456) -> (length=w463:i32)
        n231 = String Subset(string=w456, length (rest)=2 ("length (rest)")) -> (substring=w468:string)  [unwired: 1 in]
        n232 = String Subset(string=w456, length (rest)=4 ("length (rest)")) -> (substring=w466:string)  [unwired: 1 in]
        n233 = String Subset(string=w456, length (rest)=10 ("length (rest)")) -> (substring=w454:string)  [unwired: 1 in]
        n234 = Less Or Equal?(x=w463, y=0) -> (x <= y?=w460:bool)
        "x <= y?" <- w460
        n235 = Equal?(x=w466, y="Wait") -> (x = y?=w464:bool)
        n236 = Equal?(x=w468, y="Ch") -> (x = y?=w469:bool)
        n237 = Equal?(x=w454, y="Desontter ") -> ()  [unwired: 1 out]
        n238 = case shown="False" w460 {
          tunnel: w479 -> [w492 _]
          tunnel: w478 -> [w491 w557]
          tunnel: w477 -> [w490 _]
          tunnel: w458 -> [w489 _]
          tunnel: w459 -> [w488 _]
          tunnel: [w487 w557] -> w476
          tunnel: [w486 w558] -> w475
          tunnel: w474 -> [w485 w558]
          tunnel: w469 -> [w484 _]
          tunnel: w464 -> [w483 _]
          tunnel: enum32{"Output", "Input"}."Output" ("y") -> [w482 _]
          tunnel: w459 -> [w481 _]
          tunnel: w458 -> [w480 _]
          frame False {
            n239 = case shown="False" w483 {
              tunnel: w492 -> [w511 w544]
              tunnel: w491 -> [w510 w543]
              tunnel: w490 -> [w509 w547]
              tunnel: w489 -> [w508 w546]
              tunnel: w488 -> [w507 w545]
              tunnel: [w506 w542] -> w487
              tunnel: [w505 w541] -> w486
              tunnel: w485 -> [w499 _]
              tunnel: w484 -> [w498 _]
              tunnel: w482 -> [w496 _]
              tunnel: w481 -> [w494 _]
              tunnel: w480 -> [w493 _]
              frame False {
                n240 = call "DO Control.vi"("DI List_280"=w493, "s"=w498, "Control"=w494) -> ("Feedback"=w501:i32[], "Parameter (Out)"=w502:u8, "Control Channel"=w504:i32[], "Poll Time (Out)"=w503:u32, "Tab Control 2"=w495:enum32{"Output", "Input"}, "Cancel"=w497:bool)  [unwired: 3 in]
                n241 = Equal?(x=w495, y=w496) -> (x = y?=w500:bool)
                n242 = case shown="False" w497 {
                  tunnel: w511 -> [w536 _]
                  tunnel: w510 -> [w535 w538]
                  tunnel: w509 -> [w534 _]
                  tunnel: w508 -> [w533 _]
                  tunnel: w507 -> [w532 _]
                  tunnel: [w531 w538] -> w506
                  tunnel: [w530 w539] -> w505
                  tunnel: w504 -> [w521 _]
                  tunnel: w503 -> [w520 _]
                  tunnel: w502 -> [w519 _]
                  tunnel: w501 -> [w518 _]
                  tunnel: w500 -> [w512 _]
                  tunnel: w499 -> [_ w539]
                  frame False {
                    n243 = property on="Feature List" class="MCListbox (strict)"() -> ("Value"=w522:i32)  [unwired: 2 in, 2 out]
                    n244 = Index Array(array=w535, index=w522) -> (element=w527:T21)
                    n245 = Select(t="C", s=w512, f="F") -> (s? t:f=w515:string)
                    n246 = Select(t=w521, s=w512, f=w518) -> (s? t:f=w514:i32[])
                    n247 = disable-structure shown="Disabled" {
                      disable-tunnel: w512 -> [w537 _]
                      frame Disabled {
                        n248 = call "Configuration-PromptForChannelParameters_timer.vi"("Control/Feedback\n(Default: False = Feedback)"=w537) -> ()  [unwired: 13 in, 2 out]
                      }
                      frame Enabled {
                      }
                    }
                    n249 = call "ConvertNumericChannelsToStringChannels.vi"("Channels (In)"=w514) -> ("Channels (A:B:C:D...) (Out)"=w513:string)  [unwired: 14 in]
                    n250 = Unbundle By Name(w527) -> ("Steps"=w529:T22)
                    n251 = Bundle By Name(cluster=w536, "Channel Type"=w515, "Channels"=w513, "Wait/Poll (ms)"=w520, "Parameter"=w519) -> (w528:T20)
                    n252 = property on="Program step" class="LstBox (strict)"() -> ("Value"=w523:i32)  [unwired: 2 in, 2 out]
                    n253 = Replace Array Subset(array=w529, new element=w528, index=w523) -> (w525:T22)
                    n254 = Bundle By Name(cluster=w527, "Steps"=w525) -> (w526:T21)
                    n255 = call "BuildStepListFromSteps.vi"("Steps"=w525, "Control Channels"=w532, "Feedback Channels"=w533, "AI"=w534) -> ("Step List"=w530:string[])  [unwired: 11 in]
                    "Step List 2" <- w530
                    n256 = Replace Array Subset(array=w535, new element=w526, index=w522) -> (w531:T4)
                    n257 = property on="Program step" class="LstBox (strict)"("Key Focus"=TRUE, "Value"=w523, "Item Names"=w530) -> ()  [unwired: 2 in, 2 out]
                  }
                  frame True {
                  }
                }
              }
              frame True {
                n258 = property on="Feature List" class="MCListbox (strict)"() -> ("Value"=w548:i32)  [unwired: 2 in, 2 out]
                n259 = call "Timer.vi"() -> ("Wait Time out"=w540:u32)  [unwired: 10 in, 1 out]
                n260 = Index Array(array=w543, index=w548) -> (element=w552:T21)
                n261 = Bundle By Name(cluster=w544, "Channel Type"="N", "Wait/Poll (ms)"=w540) -> (w554:T20)
                n262 = Unbundle By Name(w552) -> ("Steps"=w553:T22)
                n263 = property on="Program step" class="LstBox (strict)"() -> ("Value"=w555:i32)  [unwired: 2 in, 2 out]
                n264 = Replace Array Subset(array=w553, new element=w554, index=w555) -> (w550:T22)
                n265 = Bundle By Name(cluster=w552, "Steps"=w550) -> (w551:T21)
                n266 = call "BuildStepListFromSteps.vi"("Steps"=w550, "Control Channels"=w545, "Feedback Channels"=w546, "AI"=w547) -> ("Step List"=w541:string[])  [unwired: 11 in]
                n267 = property on="Program step" class="LstBox (strict)"("Item Names"=w541, "Value"=w555, "Key Focus"=TRUE) -> ()  [unwired: 2 in, 2 out]
                n268 = Replace Array Subset(array=w543, new element=w551, index=w548) -> (w542:T4)
              }
            }
          }
          frame True {
          }
        }
      }
      event Panel Close? {
        n269 = event-data() -> ()  [unwired: 1 in, 1 out]
        n270 = event-data("Discard?"=TRUE) -> ()  [unwired: 1 in, 1 out]
      }
    }
  }
  "Error Out" <- w23
